vi "detector safety.vi"(2 "Det B type":string, 3 "Det A type":string, 4 "switches in":T1={"Oven"=TRUE, "Inj A heater"=TRUE, "Inj B heater"=TRUE, "Det A"=TRUE, "Det B"=FALSE, "Det A heater"=TRUE, "Det B heater"=FALSE}, 5 "switches prev":T1={"Oven"=TRUE, "Inj A heater"=TRUE, "Inj B heater"=TRUE, "Det A"=TRUE, "Det B"=FALSE, "Det A heater"=TRUE, "Det B heater"=FALSE}) -> (0 "Det A":bool=TRUE, 1 "switches out":T1={"Oven"=TRUE, "Inj A heater"=TRUE, "Inj B heater"=TRUE, "Det A"=TRUE, "Det B"=FALSE, "Det A heater"=TRUE, "Det B heater"=FALSE})   [LabVIEW 2012]
panel:
  # "Inj B"
  # "inj A"
  # "Oven"
  # "Det A"
  # "Det B"
  # "Detector status"
  # "Detector status"
  # "Inj B"
  # "inj A"
  # "Oven"
  # "Det A"
  # "Det B"
  # "Detector status"
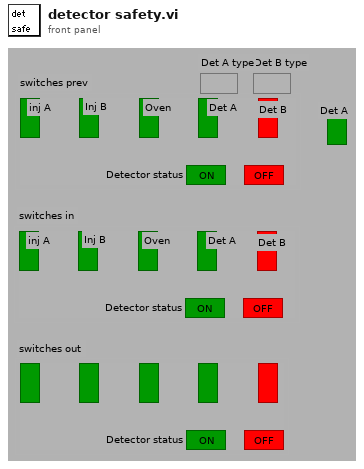
[diagram p1: front panel]
types:
  T1 = cluster{"Oven":bool, "Inj A heater":bool, "Inj B heater":bool, "Det A":bool, "Det B":bool, "Det A heater":bool, "Det B heater":bool}
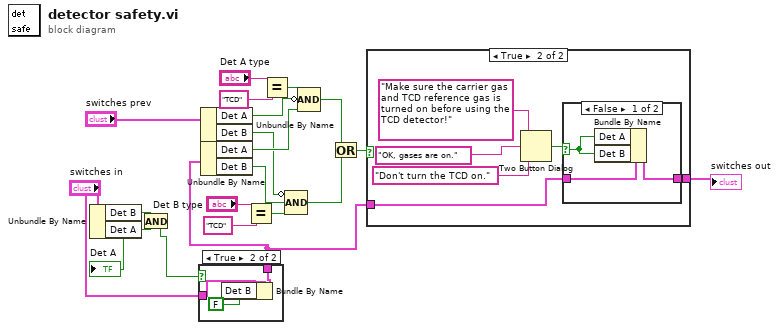
[diagram p0: block diagram]
diagram:
  n1 = Unbundle By Name("switches in") -> ("Det B"=w20:bool, "Det A"=w19:bool)
  "Det A" <- w19
  n2 = And(x=w20, y=w19) -> (x .and. y?=w18:bool)
  n3 = case shown="True" w18 {
    tunnel: [w21 w24] -> w1
    tunnel: "switches in" -> [w21 w23]
    frame False {
    }
    frame True {
      n4 = Bundle By Name(cluster=w23, "Det B"=FALSE) -> (w24:T1)
    }
  }
  n5 = Unbundle By Name("switches prev") -> ("Det A"=w13:bool, "Det B"=w7:bool)
  n6 = Unbundle By Name(w1) -> ("Det A"=w12:bool, "Det B"=w8:bool)
  n7 = Equal?(x="Det B type", y="TCD") -> (x = y?=w9:bool)
  n8 = Equal?(x="Det A type", y="TCD") -> (x = y?=w14:bool)
  n9 = Compound Arithmetic op=AND(invert w7, w8, w9) -> (w5:bool)
  n10 = Compound Arithmetic op=AND(w14, invert w13, w12) -> (w6:bool)
  n11 = Or(x=w6, y=w5) -> (x .or. y?=w4:bool)
  n12 = case shown="True" w4 {
    tunnel: [w25 w27] -> w2
    tunnel: w1 -> [w25 w26]
    frame False {
    }
    frame True {
      n13 = Two Button Dialog(message="Make sure the carrier gas and TCD reference gas is turned on before using the TCD detector!", 1:"Don't turn the TCD on.", 2:"OK, gases are on.") -> (T button?=w28:bool)
      n14 = case shown="False" w28 {
        selector: w28 -> [w32 _]
        tunnel: [w33 w35] -> w27
        tunnel: w26 -> [w34 w35]
        frame False {
          n15 = Bundle By Name(cluster=w34, "Det A"=w32, "Det B"=w32) -> (w33:T1)
        }
        frame True {
        }
      }
    }
  }
  "switches out" <- w2
